vi "习题7.1.vi"() -> ()   [LabVIEW 2017]
uses:
  <vilib>/measure/NI_MABase.lvlib
panel:
  out "XY图":cluster{"Y":dbl[], "Y":dbl[]}(graph)
  in  "frequency 2":dbl=10.0 caption="频率 2" format="%0.2p"
  in  "amplitude 2":dbl=1.0 caption="幅值 2" format="%0.2p"
  in  "相位 2":dbl format="%.2p"
  in  "frequency":dbl=10.0 caption="频率" format="%0.2p"
  in  "amplitude":dbl=1.0 caption="幅值" format="%0.2p"
  in  "phase":dbl caption="相位" format="%.2p"
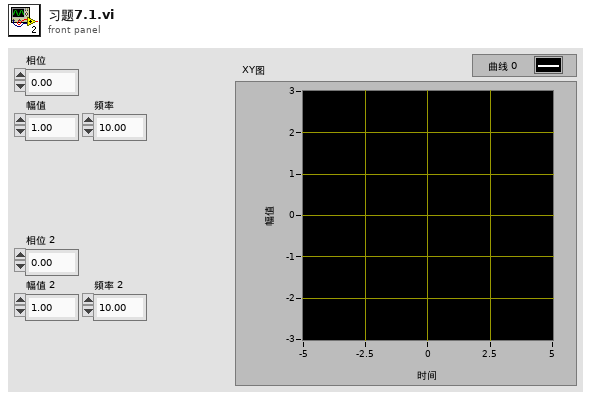
[diagram p1: front panel]
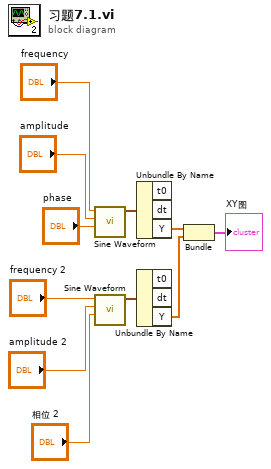
[diagram p0: block diagram]
diagram:
  n1 = call <vilib>:"Sine Waveform.vi"("phase"="phase", "amplitude"="amplitude", "frequency"="frequency") -> ("signal out"=w5:waveform(dbl))  [unwired: 7 in, 1 out]
  n2 = call <vilib>:"Sine Waveform.vi"("phase"="相位 2", "amplitude"="amplitude 2", "frequency"="frequency 2") -> ("signal out"=w4:waveform(dbl))  [unwired: 7 in, 1 out]
  n3 = Unbundle By Name(w5) -> ("Y"=w3:dbl[])  [unwired: 2 out]
  n4 = Unbundle By Name(w4) -> ("Y"=w2:dbl[])  [unwired: 2 out]
  n5 = Bundle("Y"=w3, "Y"=w2) -> (→"XY图":cluster{"Y":dbl[], "Y":dbl[]})  [unwired: 1 in]
